vi "Real Pool navigation.vi"() -> ()   [LabVIEW 2011]
uses:
  <vilib>/vision/NI_Vision_Development_Module.lvlib
panel:
  out "Boat\nHeading":sgl
  out "Boat\nLocation":cluster{"x":sgl, "y":sgl}
  out "Whale\nLocation":cluster{"x":sgl, "y":sgl}
  out "Bouy\nLocation":cluster{"x":sgl, "y":sgl}
  out "Reference\nLocation":cluster{"x":sgl, "y":sgl}
  out "Working Image":T1(plugin-control)
  out "File Type out":string
  out "File Data Type out":i32
  in  "stop":bool
  out "error out":errorcluster
  in  "Pool File Path":path=path "C:/Users/GARLAND/Documents/Projects/Robotics I/Robotics I 3390 2012/Final project/Labview/Pool navigation/pool with targets 2a.bmp"
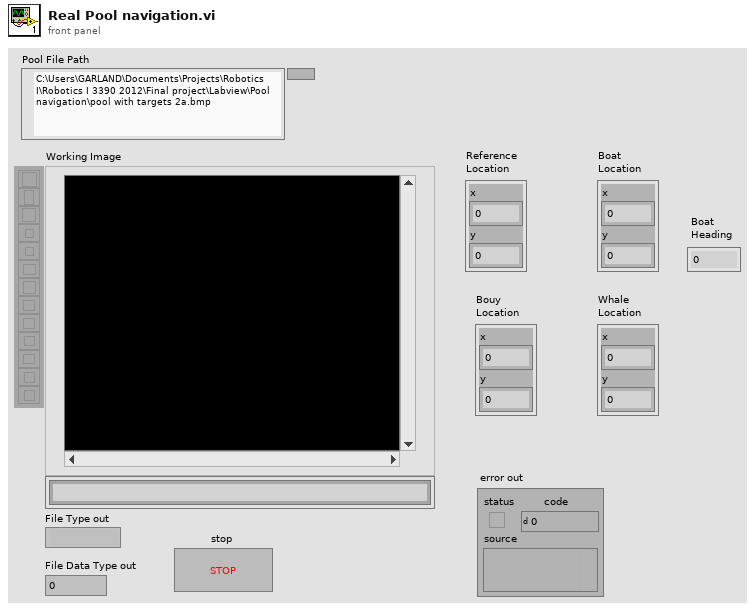
[diagram p1: front panel]
types:
  T1 = typedef "IMAQ Image.ctl" = refnum<image>
  T2 = typedef "Image Type" = u32
  T3 = cluster{"Position":cluster{"x":sgl, "y":sgl}, "Angle":sgl, "Scale":sgl, "Score":sgl, "Bounding Box":cluster{"x":sgl, "y":sgl}[]}[]
  T4 = cluster{"Position":cluster{"x":sgl, "y":sgl}, "Angle":sgl, "Scale":sgl, "Score":sgl, "Bounding Box":cluster{"x":sgl, "y":sgl}[]}
  T5 = typedef "IMAQ GM Match Report.ctl" = cluster{"Position":cluster{"x":sgl, "y":sgl}, "Angle":sgl, "Scale":sgl, "Score":sgl, "Bounding Box":cluster{"x":sgl, "y":sgl}[], "Contrast Reversed":bool, "Occlusion %":sgl, "Template Target Curve Score":sgl, "Target Template Curve Score":sgl, "Correlation Score":sgl}
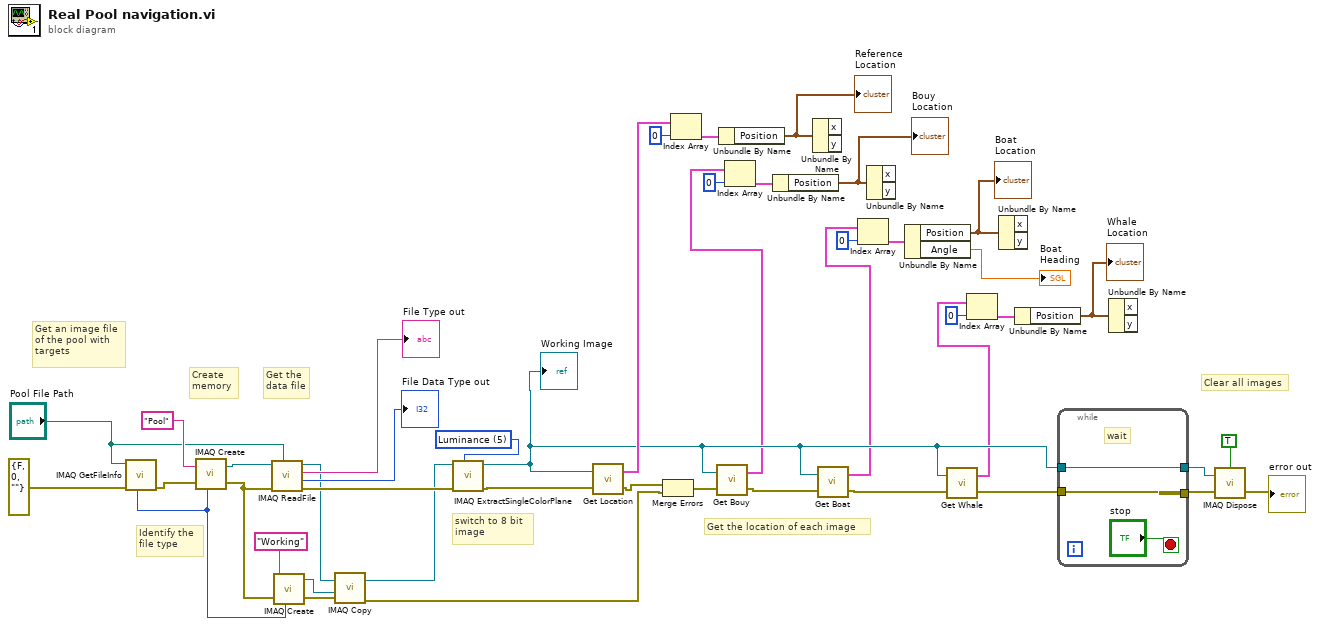
[diagram p0: block diagram]
diagram:
  w38 = 5 items=["Red", "Green", "Blue", "Hue", "Saturation", "Luminance", "Value", "Intensity"] ("Color Plane")
  # "Get the location of each image"
  # "Clear all images"
  # "switch to 8 bit \nimage"
  # "Get the \ndata file"
  # "Create \nmemory"
  # "Identify the \nfile type"
  # "Get an image file\nof the pool with\ntargets"
  n1 = call "IMAQ GetFileInfo"("error in (no error)"=errorcluster {"status"=FALSE, "code"=0, "source"=""}, "File Path"="Pool File Path") -> ("error out"=w45:errorcluster, "Image Type"=w7:T2)  [unwired: 3 in, 5 out]
  n2 = call "IMAQ Create"("Image Name"="Pool", "Image Type"=w7, "error in (no error)"=w45) -> ("New Image"=w37:T1, "error out"=w9:errorcluster)  [unwired: 2 in]
  n3 = call "IMAQ ReadFile"("File Path"="Pool File Path", "error in (no error)"=w9, "Image"=w37) -> ("error out"=w13:errorcluster, "File Data Type out"=→"File Data Type out":i32, "File Type out"=→"File Type out":string, "Image Out"=w5:T1)  [unwired: 4 in, 1 out]
  n4 = call "IMAQ Create"("Image Name"="Working", "Image Type"=w7, "error in (no error)"=w9) -> ("New Image"=w6:T1, "error out"=w10:errorcluster)  [unwired: 2 in]
  n5 = call "IMAQ Copy"("error in (no error)"=w10, "Image Dst"=w6, "Image Src"=w5) -> ("error out"=w3:errorcluster, "Image Dst Out"=w4:T1)  [unwired: 3 in]
  n6 = call "IMAQ ExtractSingleColorPlane"("Color Plane"=w38, "error in (no error)"=w13, "Image Src"=w4) -> ("error out"=w33:errorcluster, "Image Dst Out"=w26:T1)  [unwired: 1 in, 6 out]
  "Working Image" <- w26
  n7 = call "Get Location.vi"("error in"=w33, "Image"=w26) -> ("error out"=w2:errorcluster, "Matches"=w29:T3)
  n8 = Merge Errors(w2, w3) -> (w1:errorcluster)
  n9 = Index Array(array=w29, index=0) -> (element=w27:T4)
  n10 = call "Get Bouy.vi"("error in"=w1, "Image"=w26) -> ("error out"=w35:errorcluster, "Matches"=w21:T5[])
  n11 = Unbundle By Name(w27) -> ("Position"=w25:cluster{"x":sgl, "y":sgl})
  "Reference\nLocation" <- w25
  n12 = Index Array(array=w21, index=0) -> (element=w23:T5)
  n13 = Unbundle By Name(w23) -> ("Position"=w22:cluster{"x":sgl, "y":sgl})
  "Bouy\nLocation" <- w22
  n14 = Unbundle By Name(w25) -> ()  [unwired: 2 out]
  n15 = call "Get Boat.vi"("error in"=w35, "Image"=w26) -> ("error out"=w34:errorcluster, "Matches"=w18:T3)
  n16 = Index Array(array=w18, index=0) -> (element=w19:T4)
  n17 = Unbundle By Name(w22) -> ()  [unwired: 2 out]
  n18 = Unbundle By Name(w19) -> ("Position"=w12:cluster{"x":sgl, "y":sgl}, "Angle"=→"Boat\nHeading":sgl)
  "Boat\nLocation" <- w12
  n19 = call "Get Whale.vi"("error in"=w34, "Image"=w26) -> ("error out"=w32:errorcluster, "Matches"=w14:T3)
  n20 = Index Array(array=w14, index=0) -> (element=w16:T4)
  n21 = Unbundle By Name(w12) -> ()  [unwired: 2 out]
  n22 = Unbundle By Name(w16) -> ("Position"=w15:cluster{"x":sgl, "y":sgl})
  "Whale\nLocation" <- w15
  n23 = while {
    tunnel: w26 -> [w46]
    tunnel: w32 -> [w47]
    tunnel: [w47] -> w43
    tunnel: [w46] -> w31
    stop <- "stop" stop-if-true
    # "wait"
  }
  n24 = Unbundle By Name(w15) -> ()  [unwired: 2 out]
  n25 = call "IMAQ Dispose"("All Images? (No)"=TRUE, "Image"=w31, "error in (no error)"=w43) -> ("error out"=→"error out":errorcluster)  [unwired: 3 in]
